vi "oval_calcCost.vi"(8 "Error In":errorcluster, 10 "Data":variant, 11 "Elements":T1[](array[typedef])) -> (0 "Error Out":errorcluster, 3 "Elements out":T1[](array[typedef]))   [LabVIEW 2016]
uses:
  UserLibraries/AlgoritmoGenetico/TypeDefs/element.ctl
  PipePoints.ctl
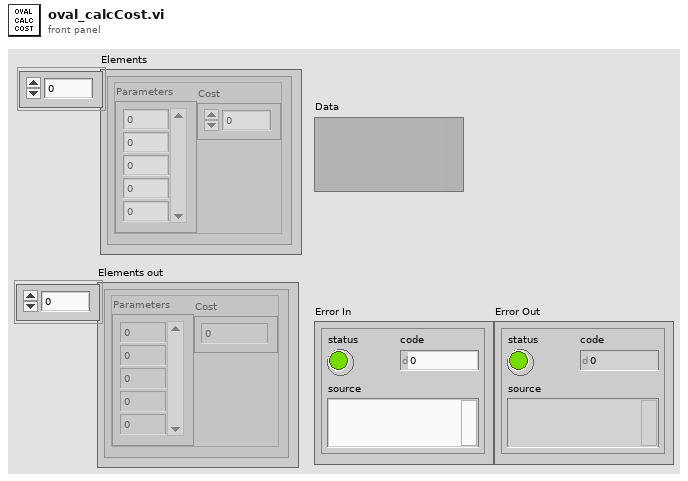
[diagram p1: front panel]
types:
  T1 = typedef "element.ctl" = cluster{"Parameters":dbl[], "Cost":dbl}
  T2 = typedef "PipePoints.ctl" = cluster{"X":dbl[], "Y":dbl[], "Theta":dbl[]}
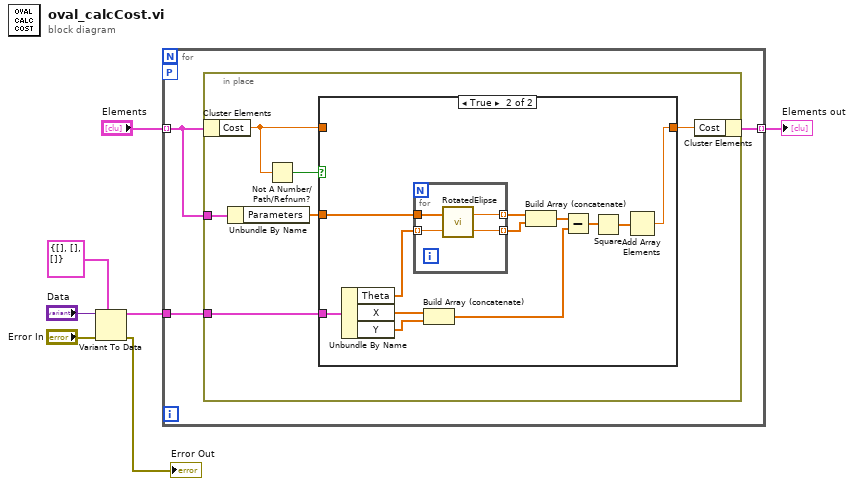
[diagram p0: block diagram]
diagram:
  n1 = Variant To Data(error in="Error In", type=T2 {"X"=[], "Y"=[], "Theta"=[]} ("PipePoints"), Variant="Data") -> (data=w1:T2, error out=→"Error Out":errorcluster)
  n2 = for {
    workers-P: _ -> [_]
    tunnel: "Elements" -> [w9] mode=indexing
    tunnel: [w10] -> w6 mode=indexing
    tunnel: w1 -> [w8]
    n3 = in-place {
      in-place-border: w9 -> [w13]
      in-place-border: w8 -> [w11]
      n4 = in-place-cluster #1(w9) -> ("Cost"=w15:dbl)
      n5 = Unbundle By Name(w13) -> ("Parameters"=w12:dbl[])
      n6 = Not A Number/Path/Refnum?(number/path/refnum=w15) -> (NaN/Path/Refnum?=w16:bool)
      n7 = case shown="True" w16 {
        tunnel: w15 -> [w17 _]
        tunnel: [w17 w18] -> w14
        tunnel: w12 -> [_ w29]
        tunnel: w11 -> [_ w28]
        frame False {
        }
        frame True {
          n8 = Unbundle By Name(w28) -> ("Theta"=w27:dbl[], "X"=w26:dbl[], "Y"=w25:dbl[])
          n9 = for {
            tunnel: w29 -> [w33]
            tunnel: w27 -> [w32] mode=indexing
            tunnel: [w31] -> w21 mode=indexing
            tunnel: [w30] -> w20 mode=indexing
            n10 = call "RotatedElipse.vi"("theta"=w32, "Parameters"=w33) -> ("y out"=w30:dbl, "x out"=w31:dbl)
          }
          n11 = Build Array (concatenate)(w26, w25) -> (w19:dbl[])
          n12 = Build Array (concatenate)(w21, w20) -> (w22:dbl[])
          n13 = Subtract(x=w22, y=w19) -> (x-y=w24:dbl[])
          n14 = Square(x=w24) -> (x^2=w23:dbl[])
          n15 = Add Array Elements(numeric array=w23) -> (sum=w18:dbl)
        }
      }
      n16 = in-place-cluster #1("Cost"=w14) -> (w10:T1)
    }
  }
  "Elements out" <- w6
